vi "dt_global.vi"() -> ()   [LabVIEW 2013]
panel:
  in  "dt":dbl
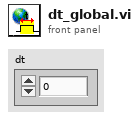
[diagram p1: front panel]
diagram:
